vi "png to pixmap.vi"(10 "Path":path) -> (0 "error out":errorcluster, 1 "Colors":u32[](array[numeric]), 2 "image":u8[](array[numeric]), 3 "path to png":path, 5 "PnG picture":picture)   [LabVIEW 2023]
doc: "Automatically finds the png file in the current VI path."
panel:
  out "appended path":path
  out "stripped path 2":path
  out "name 2":string
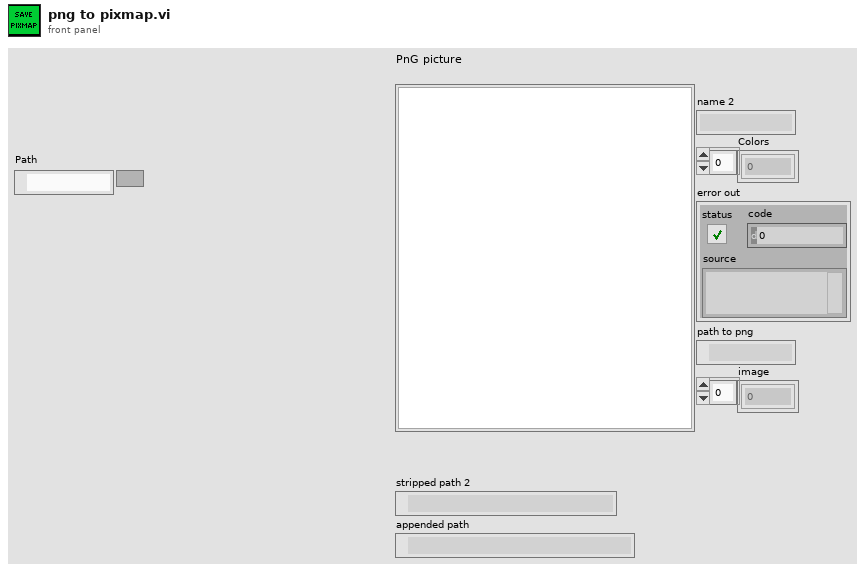
[diagram p1: front panel]
types:
  T1 = enum16{"big-endian, network order", "native, host order", "little-endian"}
  T2 = typedef "imagedata.ctl" = cluster{"image type":i32, "image depth":i32, "image":u8[], "mask":u8[], "colors":u32[], "Rectangle":cluster{"left":i16, "top":i16, "right":i16, "bottom":i16}}
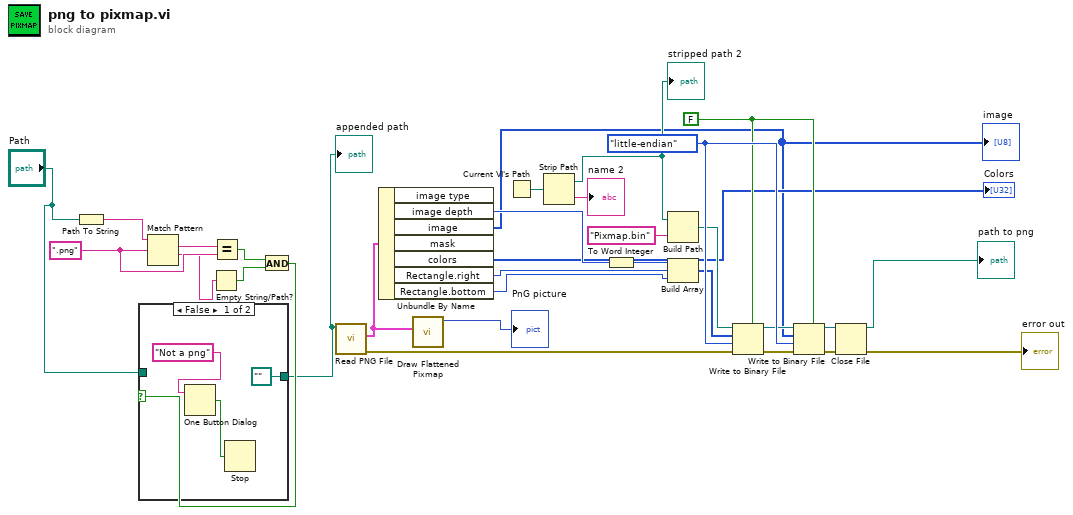
[diagram p0: block diagram]
diagram:
  w7 = ".png" ("regular expression")
  w29 = FALSE ("prepend array or string size? (T)")
  w30 = T1."little-endian" ("byte order (0:big-endian, network order)")
  n1 = Path To String(path="Path") -> (string=w9:string)
  n2 = Match Pattern(string=w9, regular expression=w7) -> (match substring=w8:string, after substring=w6:string)  [unwired: 1 in, 2 out]
  n3 = Empty String/Path?(string/path=w6) -> (empty?=w5:bool)
  n4 = Equal?(x=w8, y=w7) -> (x = y?=w4:bool)
  n5 = And(x=w4, y=w5) -> (x .and. y?=w3:bool)
  n6 = case shown="False" w3 {
    tunnel: "Path" -> [_ w36]
    tunnel: [path "" ("Path") w36] -> w1
    frame False {
      n7 = One Button Dialog(message="Not a png") -> (true=w34:bool)  [unwired: 1 in]
      n8 = Stop(stop? (T)=w34) -> ()
    }
    frame True {
    }
  }
  "appended path" <- w1
  n9 = call <vilib>:"Read PNG File.vi"("path to PNG file"=w1) -> ("error out"=w22:errorcluster, "image data"=w31:T2)  [unwired: 8 in, 1 out]
  n10 = Unbundle By Name(w31) -> ("image depth"=w19:i32, "image"=w10:u8[], "colors"=→"Colors":u32[], "Rectangle.right"=w17:i16, "Rectangle.bottom"=w16:i16)  [unwired: 2 out]
  "image" <- w10
  n11 = call <vilib>:"Draw Flattened Pixmap.vi"("image data"=w31) -> ("new picture"=→"PnG picture":picture)  [unwired: 8 in]
  n12 = Current VI's Path() -> (path=w27:path)
  n13 = Strip Path(path=w27) -> (stripped path=w24:path, name=→"name 2":string)
  "stripped path 2" <- w24
  n14 = To Word Integer(number=w19) -> (16bit integer=w18:i16)
  n15 = Build Path(base path=w24, name or relative path="Pixmap.bin") -> (appended path=w15:path)
  n16 = Build Array(w18, w17, w16) -> (w20:i16[])
  n17 = Write to Binary File(file (use dialog)=w15, data=w20, error in=w22, 5:w29, 9:w30) -> (refnum out=w14:refnum<file>, error out=w23:errorcluster)  [unwired: 1 in, 1 out]
  n18 = Write to Binary File(file (use dialog)=w14, data=w10, error in=w23, 5:w29, 9:w30) -> (refnum out=w28:refnum<file>, error out=w21:errorcluster)  [unwired: 1 in, 1 out]
  n19 = Close File(refnum=w28, error in=w21) -> (path=→"path to png":path, error out=→"error out":errorcluster)
